vi "PH_PILS.PC _TristateEOLike.vi"(0 "i ref in":refnum<vi>, 2 "serviceName":string, 3 "Value":i32, 5 "error IO":errorcluster) -> (14 "i ref out":refnum<vi>, 19 "error out":errorcluster)   [LabVIEW 2014, in "PH_PILS.lvlib"]
uses:
  PH_PILS.lvlib
  PH_Basics/PH_Common/PH_Common.lvlib
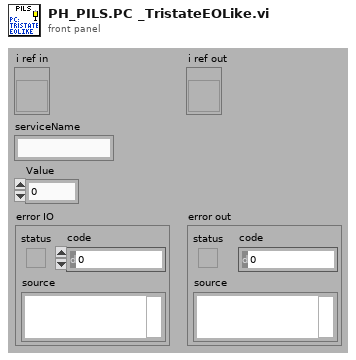
[diagram p1: front panel]
types:
  T1 = typedef "PH_PILS.lvlib/PH_PILS.i attribute.ctl" = cluster{"Boolean":cluster{"GUI Ref":refnum<vi>, "Status":i32}[], "GUI Refs Exp. Shutters":cluster{"1":refnum<vi>, "2":refnum<vi>, "3":refnum<vi>, "4":refnum<vi>}, "Tristate2Run GUI Refs":refnum<vi>[], "EO-Likes":cluster{"GUI Ref":refnum<vi>, "Status":i32}[], "Operation Mode":cluster{"Operation Mode":T2, "GUI":cluster{"Ref State":refnum<vi>, "Ref":refnum<vi>}, "Servicemode":cluster{"Tagname":string, "Status":i32}, "Labormode":cluster{"Tagname":string, "Status":i32}, "Searchmode":cluster{"Tagname":string, "Status":i32}, "Shotmode":cluster{"Tagname":string, "Status":i32}}, "Submode":cluster{"Submode":T3, "GUI":cluster{"Ref State":refnum<vi>, "Ref":refnum<vi>}, "Submode":cluster{"Tagname":string, "Status":i32}}, "Experiment":cluster{"Experiment":enum16{"unknown", "intern", "4 (Z6)", "3", "2", "1"}, "GUI":cluster{"Ref State":refnum<vi>, "Ref":refnum<vi>}, "intern":cluster{"Tagname":string, "Status":i32}, "Exp 4":cluster{"Tagname":string, "Status":i32}, "Exp 3":cluster{"Tagname":string, "Status":i32}, "Exp 2":cluster{"Tagname":string, "Status":i32}, "Exp 1":cluster{"Tagname":string, "Status":i32}}, "TristateNormal":cluster{"GUI Ref":refnum<vi>, "Status":i32}[], "Door Tags":cluster{"GUI Ref":refnum<vi>, "Status":i32}[], "GUIlessTags":cluster{"Name":string, "Status":i32}[], "Beamline GUI Refs":refnum<vi>[], "Special Boolean":cluster{"GUI Ref":refnum<vi>, "Status":i32}[], "Laserpower":cluster{"GUI Ref":refnum<vi>, "Status":i32}[], "Shutter":cluster{"GUI Ref":refnum<vi>, "Status":i32}[], "Tristate EO Like":cluster{"GUI Ref":refnum<vi>, "Status":i32}[], "PP":cluster{"GUI Ref":refnum<vi>, "Status":i32, "Head Ref":refnum<vi>, "Slider Ref":refnum<vi>}[], "Switch Knobs":cluster{"GUI Ref":refnum<vi>, "Status":i32}[], "Latch Knob GUI Refs":refnum<vi>[], "FailureCounter":i32, "Enabled Status":cluster{"Laser":i32, "PreAmp":i32, "MainAmp":i32}, "Mercury":refnum<vi>, "Instance Rods":string, "Logfile":path, "Beckhoff-Instance Internal":string, "Beckhoff-Instance External":string, "Enabling Rights":cluster{"Name":string, "Password":string, "PA?":bool, "MA?":bool, "Exp?":bool}[]}
  T2 = typedef "PH_PILS.lvlib/PH_PILS.Operation Mode.ctl" = enum16{"unknown", "Service", "Labor", "Search", "Shot"}
  T3 = typedef "PH_PILS.lvlib/PH_PILS.Submode.ctl" = enum16{"unknown", "HV-Normal", "HV-Test"}
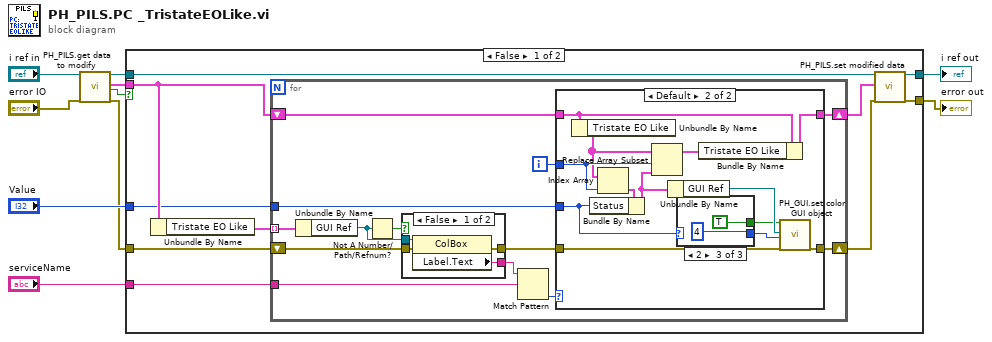
[diagram p0: block diagram]
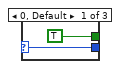
[diagram p3: hidden frame]
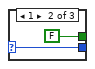
[diagram p4: hidden frame]
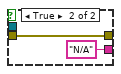
[diagram p5: hidden frame]
diagram:
  n1 = call "PH_PILS.get data to modify.vi"("i ref in"="i ref in", "error in (no error)"="error IO") -> ("i ref out"=w4:refnum<vi>, "i attribute"=w5:T1, "timed out"=w1:bool, "error out"=w6:errorcluster)  [unwired: 14 in]
  n2 = case shown="False" w1 {
    tunnel: "Value" -> [w12 _]
    tunnel: "serviceName" -> [w14 _]
    tunnel: w6 -> [w15 w61]
    tunnel: w5 -> [w17 _]
    tunnel: w4 -> [w20 w62]
    tunnel: [w19 w62] -> w3
    tunnel: [w18 w61] -> w2
    frame False {
      n3 = Unbundle By Name(w17) -> ("Tristate EO Like"=w13:cluster{"GUI Ref":refnum<vi>, "Status":i32}[])
      n4 = for {
        tunnel: w13 -> [w33] mode=indexing
        shift-right: [w26] -> w11
        shift-left: w15 -> [w32]
        tunnel: w14 -> [w21]
        shift-right: [w24] -> w16
        shift-left: w17 -> [w25]
        tunnel: w12 -> [w23]
        i -> [w28]
        n5 = Unbundle By Name(w33) -> ("GUI Ref"=w30:refnum<vi>)
        n6 = Not A Number/Path/Refnum?(number/path/refnum=w30) -> (NaN/Path/Refnum?=w31:bool)
        n7 = case shown="False" w31 {
          tunnel: w30 -> [w58 _]
          tunnel: w32 -> [w57 w60]
          tunnel: [w56 w60] -> w27
          tunnel: [w55 "N/A" ("Label.Text")] -> w22
          frame False {
            n8 = property class="ColBox"(reference=w58, error in=w57) -> (error out=w56:errorcluster, "Label.Text"=w55:string)  [unwired: 1 out]
          }
          frame True {
          }
        }
        n9 = Match Pattern(string=w22, regular expression=w21) -> (offset past match=w29:i32)  [unwired: 1 in, 3 out]
        n10 = case shown="Default" w29 {
          tunnel: w27 -> [w34 w48]
          tunnel: [w34 w47] -> w26
          tunnel: w25 -> [w35 w42]
          tunnel: [w35 w46] -> w24
          tunnel: w23 -> [_ w38]
          tunnel: w28 -> [_ w43]
          frame -1 {
          }
          frame Default {
            n11 = Unbundle By Name(w42) -> ("Tristate EO Like"=w41:cluster{"GUI Ref":refnum<vi>, "Status":i32}[])
            n12 = Index Array(array=w41, index=w43) -> (element=w44:cluster{"GUI Ref":refnum<vi>, "Status":i32})
            n13 = Bundle By Name(cluster=w44, "Status"=w38) -> (w40:cluster{"GUI Ref":refnum<vi>, "Status":i32})
            n14 = Replace Array Subset(array=w41, new element=w40, index=w43) -> (w45:cluster{"GUI Ref":refnum<vi>, "Status":i32}[])
            n15 = Unbundle By Name(w40) -> ("GUI Ref"=w39:refnum<vi>)
            n16 = case shown="2" w38 {
              selector: w38 -> [w50 w51 _]
              tunnel: [w50 w51 4 ("Value")] -> w37
              tunnel: [TRUE FALSE TRUE] -> w36
              frame 0, Default {
              }
              frame 1 {
              }
              frame 2 {
              }
            }
            n17 = Bundle By Name(cluster=w42, "Tristate EO Like"=w45) -> (w46:T1)
            n18 = call "PH_GUI.set color GUI object.vi"("Visible? (true)"=w36, "GUI object Ref"=w39, "State"=w37, "error in (no error)"=w48) -> ("error out"=w47:errorcluster)  [unwired: 15 in]
          }
        }
      }
      n19 = call "PH_PILS.set modified data.vi"("i ref in"=w20, "i attribute"=w16, "error in (no error)"=w11) -> ("i ref out"=w19:refnum<vi>, "error out"=w18:errorcluster)  [unwired: 15 in]
    }
    frame True {
    }
  }
  "error out" <- w2
  "i ref out" <- w3
